vi "debugger File Speed.vi"(8 "error in (no error)":errorcluster, 9 "Empty Results":T1={"Measurement Cycles"=1, "Measurement Values"={"Rab (ohms)"=615.28, "Rac (ohms)"=30.6972, "Rbc (ohms)"=399.129, "Zo (ohms)"=0.0, "Attenuation (dB)"=inf, "Zin (ohms)"=9.15444, "Zout (ohms)"=119.027, "R1 (ohms)"=-39.4037, "R2 (ohms)"=7.4286, "R3 (ohms)"=29.6035}, "Topology"=enum."PI-Network", "DCA_Status"=TRUE, "Limits and Passed?"={"Limits"=[], "Passed? Array"=[]}, "Normalization"={"Normalized?"=FALSE, "Rab Value"=0.0, "Rac Value"=0.0, "Rbc Value"=0.0}, "ATTN Calc"=enum."Power", "Instruments to Use"={"DMM Instrument Record"={"ixInstrument"=0, "sxInstrumentId"="", "sDriverId"="", "sDriverType"="", "sSerialNumber"="", "tLastCalibration"=timestamp(0 s since 1904-01-01), "tCalibrationDue"=timestamp(0 s since 1904-01-01), "sConfiguration"=""}, "SWI Instrument Record"={"ixInstrument"=0, "sxInstrumentId"="", "sDriverId"="", "sDriverType"="", "sSerialNumber"="", "tLastCalibration"=timestamp(0 s since 1904-01-01), "tCalibrationDue"=timestamp(0 s since 1904-01-01), "sConfiguration"=""}}}, 10 "Fields":T12[](array[typedef])=[{"ixField"=14420, "iSequenceOrder"=0, "sxFieldId"="Serial_Number", "sxSequenceId"="Debugger File Speed", "sDisplayName"="Serial Number", "sValue"="Debugger File Speed", "sUnits"="", "nDataType"=enum."text", "nNextItem"=enum."Reset", "fSystem"=TRUE, "fSystemValue"=FALSE, "fRequired"=TRUE, "fSetAtTest"=FALSE, "fTestField"=FALSE, "fDeleted"=FALSE, "fIndexed"=TRUE, "fFreeList"=FALSE}, {"ixField"=14825, "iSequenceOrder"=0, "sxFieldId"="Test_Version", "sxSequenceId"="Debugger File Speed", "sDisplayName"="Test Version", "sValue"="  v  0000", "sUnits"="", "nDataType"=enum."timestamp", "nNextItem"=enum."Reset", "fSystem"=FALSE, "fSystemValue"=FALSE, "fRequired"=FALSE, "fSetAtTest"=FALSE, "fTestField"=FALSE, "fDeleted"=FALSE, "fIndexed"=FALSE, "fFreeList"=FALSE}, {"ixField"=14421, "iSequenceOrder"=0, "sxFieldId"="Model_Number", "sxSequenceId"="Debugger File Speed", "sDisplayName"="Model Number", "sValue"="Debugger File Speed", "sUnits"="", "nDataType"=enum."timestamp", "nNextItem"=enum."Reset", "fSystem"=TRUE, "fSystemValue"=FALSE, "fRequired"=TRUE, "fSetAtTest"=FALSE, "fTestField"=FALSE, "fDeleted"=FALSE, "fIndexed"=TRUE, "fFreeList"=FALSE}, {"ixField"=14422, "iSequenceOrder"=0, "sxFieldId"="Test_Run", "sxSequenceId"="Debugger File Speed", "sDisplayName"="Test Run", "sValue"="1", "sUnits"="", "nDataType"=enum."timestamp", "nNextItem"=enum."Reset", "fSystem"=FALSE, "fSystemValue"=FALSE, "fRequired"=FALSE, "fSetAtTest"=FALSE, "fTestField"=FALSE, "fDeleted"=FALSE, "fIndexed"=FALSE, "fFreeList"=FALSE}, {"ixField"=14423, "iSequenceOrder"=0, "sxFieldId"="Start_Timestamp", "sxSequenceId"="Debugger File Speed", "sDisplayName"="Start Timestamp", "sValue"="3284394075.382834", "sUnits"="", "nDataType"=enum."timestamp", "nNextItem"=enum."Reset", "fSystem"=FALSE, "fSystemValue"=FALSE, "fRequired"=FALSE, "fSetAtTest"=FALSE, "fTestField"=FALSE, "fDeleted"=FALSE, "fIndexed"=FALSE, "fFreeList"=FALSE}, {"ixField"=14424, "iSequenceOrder"=0, "sxFieldId"="End_Timestamp", "sxSequenceId"="Debugger File Speed", "sDisplayName"="End Timestamp", "sValue"="3284394080.601751", "sUnits"="", "nDataType"=enum."timestamp", "nNextItem"=enum."Reset", "fSystem"=FALSE, "fSystemValue"=FALSE, "fRequired"=FALSE, "fSetAtTest"=FALSE, "fTestField"=FALSE, "fDeleted"=FALSE, "fIndexed"=FALSE, "fFreeList"=FALSE}, {"ixField"=14425, "iSequenceOrder"=0, "sxFieldId"="Test_Status", "sxSequenceId"="Debugger File Speed", "sDisplayName"="Test Status", "sValue"="Fail", "sUnits"="", "nDataType"=enum."timestamp", "nNextItem"=enum."Reset", "fSystem"=FALSE, "fSystemValue"=FALSE, "fRequired"=FALSE, "fSetAtTest"=FALSE, "fTestField"=FALSE, "fDeleted"=FALSE, "fIndexed"=FALSE, "fFreeList"=FALSE}, {"ixField"=14426, "iSequenceOrder"=0, "sxFieldId"="Test_Type", "sxSequenceId"="Debugger File Speed", "sDisplayName"="Test Type", "sValue"="DC Attenuation", "sUnits"="", "nDataType"=enum."timestamp", "nNextItem"=enum."Reset", "fSystem"=FALSE, "fSystemValue"=FALSE, "fRequired"=FALSE, "fSetAtTest"=FALSE, "fTestField"=FALSE, "fDeleted"=FALSE, "fIndexed"=FALSE, "fFreeList"=FALSE}, {"ixField"=14427, "iSequenceOrder"=0, "sxFieldId"="Test_Sequence", "sxSequenceId"="Debugger File Speed", "sDisplayName"="Test Sequence", "sValue"="Debugger File Speed", "sUnits"="", "nDataType"=enum."timestamp", "nNextItem"=enum."Reset", "fSystem"=FALSE, "fSystemValue"=FALSE, "fRequired"=FALSE, "fSetAtTest"=FALSE, "fTestField"=FALSE, "fDeleted"=FALSE, "fIndexed"=FALSE, "fFreeList"=FALSE}, {"ixField"=14428, "iSequenceOrder"=0, "sxFieldId"="Operator", "sxSequenceId"="Debugger File Speed", "sDisplayName"="Operator", "sValue"="Debugger File Speed", "sUnits"="", "nDataType"=enum."timestamp", "nNextItem"=enum."Reset", "fSystem"=FALSE, "fSystemValue"=FALSE, "fRequired"=FALSE, "fSetAtTest"=FALSE, "fTestField"=FALSE, "fDeleted"=FALSE, "fIndexed"=FALSE, "fFreeList"=FALSE}, {"ixField"=14430, "iSequenceOrder"=0, "sxFieldId"="Test_Station", "sxSequenceId"="Debugger File Speed", "sDisplayName"="Test Station", "sValue"="127.0.0.1", "sUnits"="", "nDataType"=enum."timestamp", "nNextItem"=enum."Reset", "fSystem"=FALSE, "fSystemValue"=FALSE, "fRequired"=FALSE, "fSetAtTest"=FALSE, "fTestField"=FALSE, "fDeleted"=FALSE, "fIndexed"=FALSE, "fFreeList"=FALSE}, {"ixField"=14431, "iSequenceOrder"=0, "sxFieldId"="Company", "sxSequenceId"="Debugger File Speed", "sDisplayName"="Company", "sValue"="Summitek Instruments", "sUnits"="", "nDataType"=enum."timestamp", "nNextItem"=enum."Reset", "fSystem"=FALSE, "fSystemValue"=FALSE, "fRequired"=FALSE, "fSetAtTest"=FALSE, "fTestField"=FALSE, "fDeleted"=FALSE, "fIndexed"=FALSE, "fFreeList"=FALSE}, {"ixField"=14432, "iSequenceOrder"=0, "sxFieldId"="Step_Number", "sxSequenceId"="Debugger File Speed", "sDisplayName"="Step Number", "sValue"="1", "sUnits"="", "nDataType"=enum."timestamp", "nNextItem"=enum."Reset", "fSystem"=FALSE, "fSystemValue"=FALSE, "fRequired"=FALSE, "fSetAtTest"=FALSE, "fTestField"=FALSE, "fDeleted"=FALSE, "fIndexed"=FALSE, "fFreeList"=FALSE}, {"ixField"=14433, "iSequenceOrder"=0, "sxFieldId"="Step_Tag", "sxSequenceId"="Debugger File Speed", "sDisplayName"="Step Tag", "sValue"="", "sUnits"="", "nDataType"=enum."timestamp", "nNextItem"=enum."Reset", "fSystem"=FALSE, "fSystemValue"=FALSE, "fRequired"=FALSE, "fSetAtTest"=FALSE, "fTestField"=FALSE, "fDeleted"=FALSE, "fIndexed"=FALSE, "fFreeList"=FALSE}], 11 "Iterations":i32=10) -> (0 "error out":errorcluster, 3 "js timing results":string="{ iterations: 10, group1: 0.000000, group2: 0.000000, chdata: 1.400000, open: 0.300000, close: 0.000000, total: 1.700000 }")   [LabVIEW 2011]
uses:
  server/database/Fields/Field Record.ctl
  server/database/Fields/Field DataTypes.ctl
  server/database/Fields/Field NextItem.ctl
  tests/DC Attenuation/TypeDefs/DCA Results.ctl
  tests/DC Attenuation/TypeDefs/DCA Measurement Values.ctl
  tests/DC Attenuation/TypeDefs/DCA Topology.ctl
  tests/DC Attenuation/TypeDefs/DCA Limit.ctl
  tests/DC Attenuation/TypeDefs/DCA Limit Quantity.ctl
  tests/DC Attenuation/TypeDefs/DCA Limit Comparison.ctl
  tests/DC Attenuation/TypeDefs/DCA Limit Operation.ctl
  tests/Test Referential Limit.ctl
  tests/DC Attenuation/TypeDefs/DCA Calibration State.ctl
  tests/DC Attenuation/TypeDefs/DCA Attenuation Calculation.ctl
  server/database/Stations/Instruments/Instrument Record.ctl
  server/database/Fields/Field System Fields.ctl
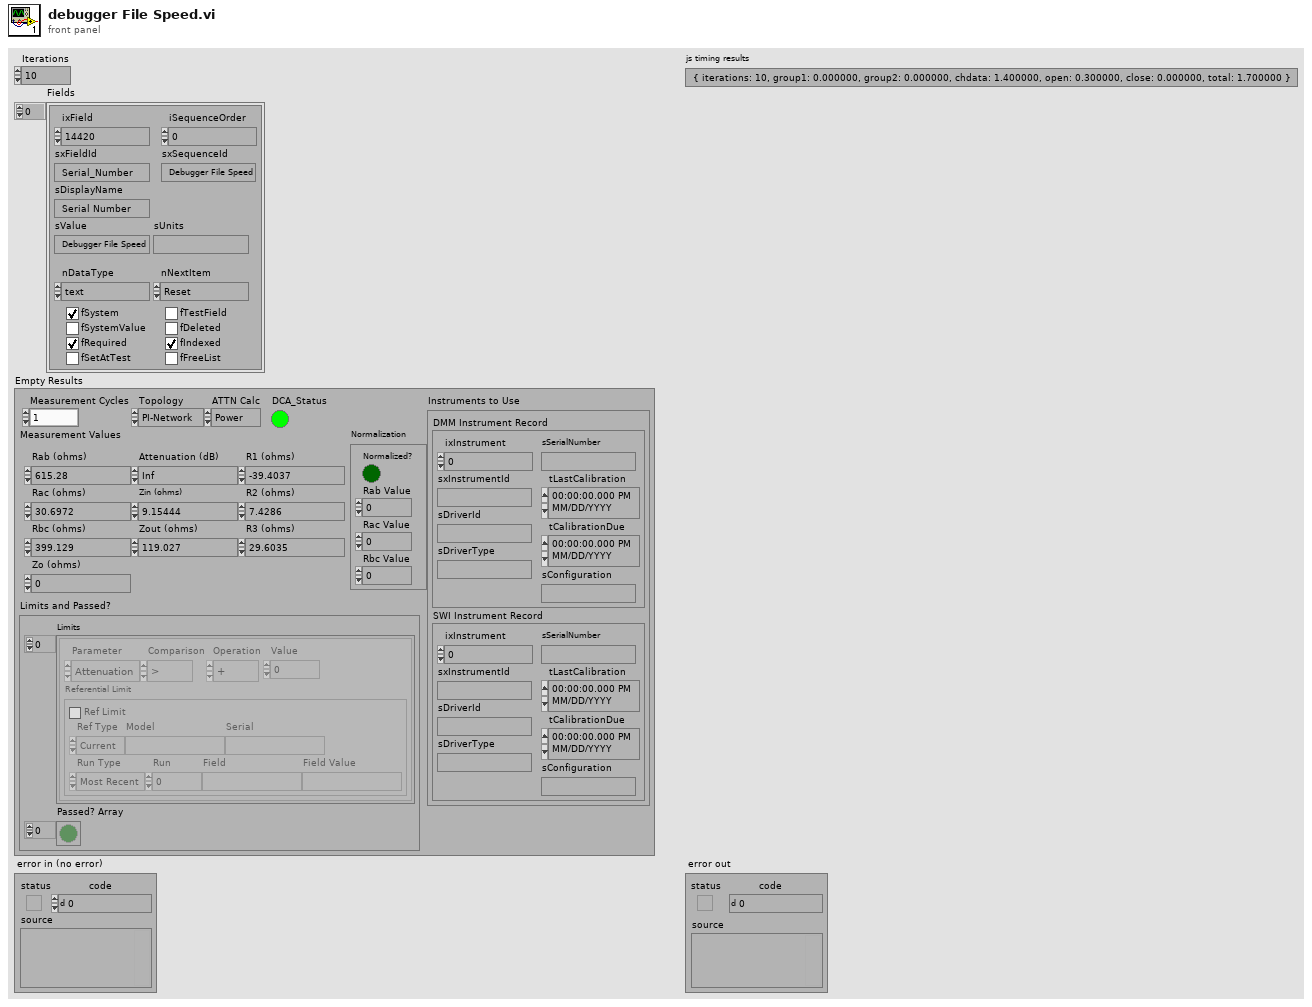
[diagram p1: front panel]
types:
  T1 = typedef "DCA Results.ctl" = cluster{"Measurement Cycles":i32, "Measurement Values":T2, "Topology":T3, "DCA_Status":bool, "Limits and Passed?":cluster{"Limits":T4[], "Passed? Array":bool[]}, "Normalization":T9, "ATTN Calc":T10, "Instruments to Use":cluster{"DMM Instrument Record":T11, "SWI Instrument Record":T11}}
  T2 = typedef "DCA Measurement Values.ctl" = cluster{"Rab (ohms)":dbl, "Rac (ohms)":dbl, "Rbc (ohms)":dbl, "Zo (ohms)":dbl, "Attenuation (dB)":dbl, "Zin (ohms)":dbl, "Zout (ohms)":dbl, "R1 (ohms)":dbl, "R2 (ohms)":dbl, "R3 (ohms)":dbl}
  T3 = typedef "DCA Topology.ctl" = enum32{"PI-Network", "T-Network"}
  T4 = typedef "DCA Limit.ctl" = cluster{"Parameter":T5, "Comparison":T6, "Operation":T7, "Value":dbl, "Referential Limit":T8}
  T5 = typedef "DCA Limit Quantity.ctl" = enum16{"Attenuation", "Zin", "Zout", "R1", "R2", "R3", "Rab", "Rac", "Rbc"}
  T6 = typedef "DCA Limit Comparison.ctl" = enum16{">", ">=", "<", "<="}
  T7 = typedef "DCA Limit Operation.ctl" = enum16{"+", "-"}
  T8 = typedef "Test Referential Limit.ctl" = cluster{"Ref Limit":bool, "Ref Type":enum16{"Current", "Specify"}, "Model":string, "Serial":string, "Run Type":enum16{"Most Recent", "Run #", "Match Field"}, "Run":i32, "Field":string, "Field Value":string}
  T9 = typedef "DCA Calibration State.ctl" = cluster{"Normalized?":bool, "Rab Value":dbl, "Rac Value":dbl, "Rbc Value":dbl}
  T10 = typedef "DCA Attenuation Calculation.ctl" = enum32{"Power", "Voltage"}
  T11 = typedef "Instrument Record.ctl" = cluster{"ixInstrument":i32, "sxInstrumentId":string, "sDriverId":string, "sDriverType":string, "sSerialNumber":string, "tLastCalibration":timestamp, "tCalibrationDue":timestamp, "sConfiguration":string}
  T12 = typedef "Field Record.ctl" = cluster{"ixField":i32, "iSequenceOrder":i32, "sxFieldId":string, "sxSequenceId":string, "sDisplayName":string, "sValue":string, "sUnits":string, "nDataType":T13, "nNextItem":T14, "fSystem":bool, "fSystemValue":bool, "fRequired":bool, "fSetAtTest":bool, "fTestField":bool, "fDeleted":bool, "fIndexed":bool, "fFreeList":bool}
  T13 = typedef "Field DataTypes.ctl" = enum32{"text", "numeric", "list", "timestamp", "boolean"}
  T14 = typedef "Field NextItem.ctl" = enum32{"Reset", "Retain", "Auto-Increment"}
  T15 = enum16{"open", "open or create", "create or replace", "create", "open (read-only)"}
  T16 = typedef "Field System Fields.ctl" = enum32{"Company", "End_Timestamp", "Model_Number", "Operator", "Serial_Number", "Start_Timestamp", "Step_Number", "Step_Tag", "Test_Run", "Test_Sequence", "Test_Station", "Test_Station_Name", "Test_Status", "Test_Type", "Test_Version", "Spartan_Version_Created", "Spartan_Version_Current"}
  T17 = typedef "TDMS Timing.ctl" = cluster{"Open\\Create":u32, "Group Properties 1":u32, "Group Properties 2":u32, "Channel Data":u32, "Close":u32, "Total":u32}
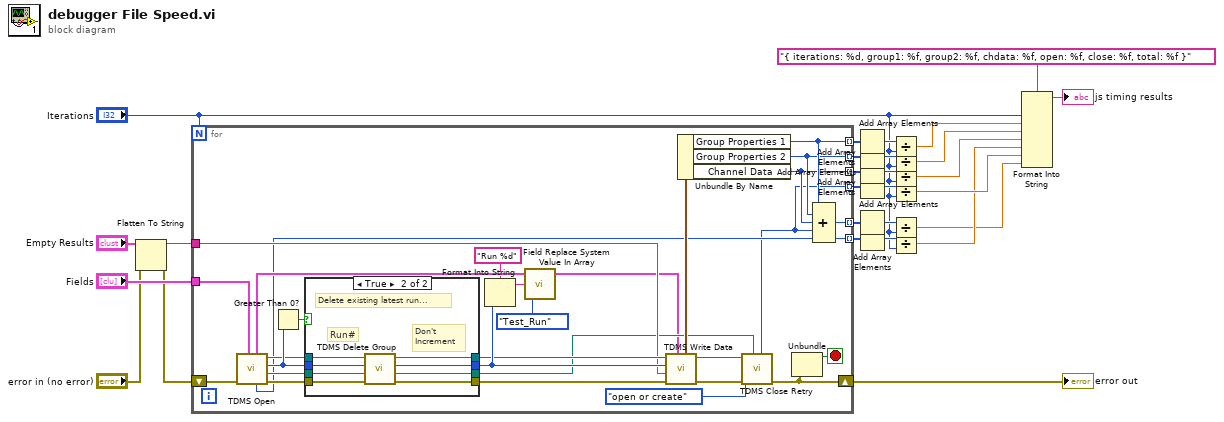
[diagram p0: block diagram]
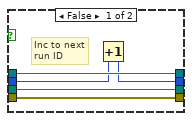
[diagram p2: hidden frame]
diagram:
  n1 = Flatten To String(anything="Empty Results", error in (no error)="error in (no error)") -> (data string=w11:string, error out=w13:errorcluster)  [unwired: 3 out]
  n2 = for {
    N: "Iterations" -> [_]
    shift-right: [w33] -> w1
    shift-left: w13 -> [w42]
    tunnel: w11 -> [w43]
    tunnel: "Fields" -> [w29]
    tunnel: [w41] -> w19 mode=indexing
    tunnel: [w40] -> w25 mode=indexing
    tunnel: [w38] -> w15 mode=indexing
    tunnel: [w37] -> w16 mode=indexing
    tunnel: [w30] -> w17 mode=indexing
    tunnel: [w36] -> w18 mode=indexing
    stop <- w39 stop-if-true
    n3 = call "TDMS Open.vi"("Fields In"=w29, "error in (no error)"=w42) -> ("error out"=w49:errorcluster, "TDMS File Path"=w52:path, "Last Run #"=w51:i32, "TDMS File Ref"=w50:refnum<k34>, "Execution Time (ms)"=w41:u32, "Fields Out"=w47:T12[])  [unwired: 1 in, 3 out]
    n4 = Greater Than 0?(x=w51) -> (x > 0?=w48:bool)
    n5 = case shown="True" w48 {
      tunnel: w49 -> [w61 w69]
      tunnel: [w61 w68] -> w53
      tunnel: w51 -> [w59 w65]
      tunnel: [w58 w62] -> w55
      tunnel: [w60 w66] -> w54
      tunnel: w50 -> [w60 w67]
      tunnel: w52 -> [w57 w64]
      tunnel: [w57 w63] -> w31
      frame False {
        # "Inc to next\nrun ID"
        n6 = Increment(x=w59) -> (x+1=w58:i32)
      }
      frame True {
        # "Don't \nIncrement"
        # "Run#"
        # "Delete existing latest run..."
        n7 = call "TDMS Delete Group.vi"("error in (no error)"=w69, "File Path In"=w64, "Run to Delete"=w65, "TDMS File Ref"=w67) -> ("error out"=w68:errorcluster, "File Path Out"=w63:path, "Run #"=w62:i32, "TDMS File Ref"=w66:refnum<k34>)  [unwired: 1 in, 3 out]
      }
    }
    n8 = Format Into String(format string="Run %d", w55) -> (resulting string=w46:string)  [unwired: 2 in, 1 out]
    n9 = call "Field Replace System Value In Array.vi"("System Field to Replace (Serial Number)"=Field_System_Fields."Test_Run", "Field Value Replacement Data (\"\")"=w46, "Fields Array In"=w47) -> ("Fields Array Out"=w28:T12[])  [unwired: 1 in, 1 out]
    n10 = call "TDMS Write Data.vi"("Fields Array In"=w28, "error in (no error)"=w53, "Test Results (\"\")"=w43, "Test Run (1)"=w55, "TDMS File Ref"=w54) -> ("error out"=w34:errorcluster, "TDMS File Ref"=w35:refnum<k34>, "Timing (ms)"=w56:T17)  [unwired: 1 in, 3 out]
    n11 = Unbundle By Name(w56) -> ("Group Properties 1"=w40:u32, "Group Properties 2"=w38:u32, "Channel Data"=w37:u32)
    n12 = call "TDMS Close Retry.vi"("TDMS Path"=w31, "error in (no error)"=w34, "Operation (0:open)"=T15."open or create", "TDMS File Ref"=w35) -> ("error out"=w33:errorcluster, "Execution Time (ms)"=w30:u32)  [unwired: 1 in, 5 out]
    n13 = Unbundle(w33) -> ("status"=w39:bool)  [unwired: 2 out]
    n14 = Compound Arithmetic op=ADD(w40, w38, w37, w30, w41) -> (w36:u32)
  }
  "error out" <- w1
  n15 = Add Array Elements(numeric array=w25) -> (sum=w26:u32)
  n16 = Add Array Elements(numeric array=w15) -> (sum=w24:u32)
  n17 = Add Array Elements(numeric array=w16) -> (sum=w23:u32)
  n18 = Add Array Elements(numeric array=w17) -> (sum=w22:u32)
  n19 = Add Array Elements(numeric array=w18) -> (sum=w21:u32)
  n20 = Add Array Elements(numeric array=w19) -> (sum=w20:u32)
  n21 = Divide(x=w26, y="Iterations") -> (x/y=w8:dbl)
  n22 = Divide(x=w24, y="Iterations") -> (x/y=w7:dbl)
  n23 = Divide(x=w23, y="Iterations") -> (x/y=w6:dbl)
  n24 = Divide(x=w22, y="Iterations") -> (x/y=w5:dbl)
  n25 = Divide(x=w21, y="Iterations") -> (x/y=w3:dbl)
  n26 = Divide(x=w20, y="Iterations") -> (x/y=w4:dbl)
  n27 = Format Into String(format string="{ iterations: %d, group1: %f, group2: %f, chdata: %f, open: %f, close: %f, total: %f }", "Iterations", w8, w7, w6, w4, w5, w3) -> (resulting string=→"js timing results":string)  [unwired: 2 in, 1 out]
